vi "Acc_Z.vi"(1 "z_ini":dbl) -> (0 "z_Acc":dbl)   [LabVIEW 2010]
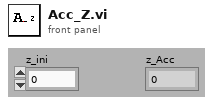
[diagram p1: front panel]
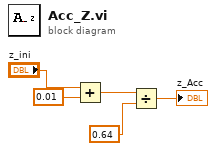
[diagram p0: block diagram]
diagram:
  n1 = Add(x="z_ini", y=0.01) -> (x+y=w3:dbl)
  n2 = Divide(x=w3, y=0.64) -> (x/y=→"z_Acc":dbl)
